vi "Build.vi"(6 "Type of Hexaboard":T1, 9 "XYZTheta":dbl[](array[numeric]), 10 "Pattern Coordinates":dbl[][](array[numeric]), 11 "C4 Dispense in":refnum<class "Iterative Dispense.lvclass">) -> (3 "C4 Dispense out":refnum<class "Iterative Dispense.lvclass">)   [LabVIEW 2021, in "Iterative Dispense.lvclass"]
uses:
  Iterative Dispense.lvclass
  C:/Users/hep/Documents/UCSB-CMU-GantryCode/UCSB-Gantry-HEP-main (3)/UCSB-Gantry-HEP-main/Classes/Routine/Dispense/Dispense.lvclass
  TypeOfHexaboard.ctl
  Iterative Dispense.lvclass/Iterative Dispense.ctl
  <vilib>/Analysis/coordinate.llb/2D Cartesian Coordinate Rotation (Array).vi
  <vilib>/Analysis/NI_AALPro.lvlib
  Routine.lvclass
panel:
  out "Array":dbl[][][](array[numeric])
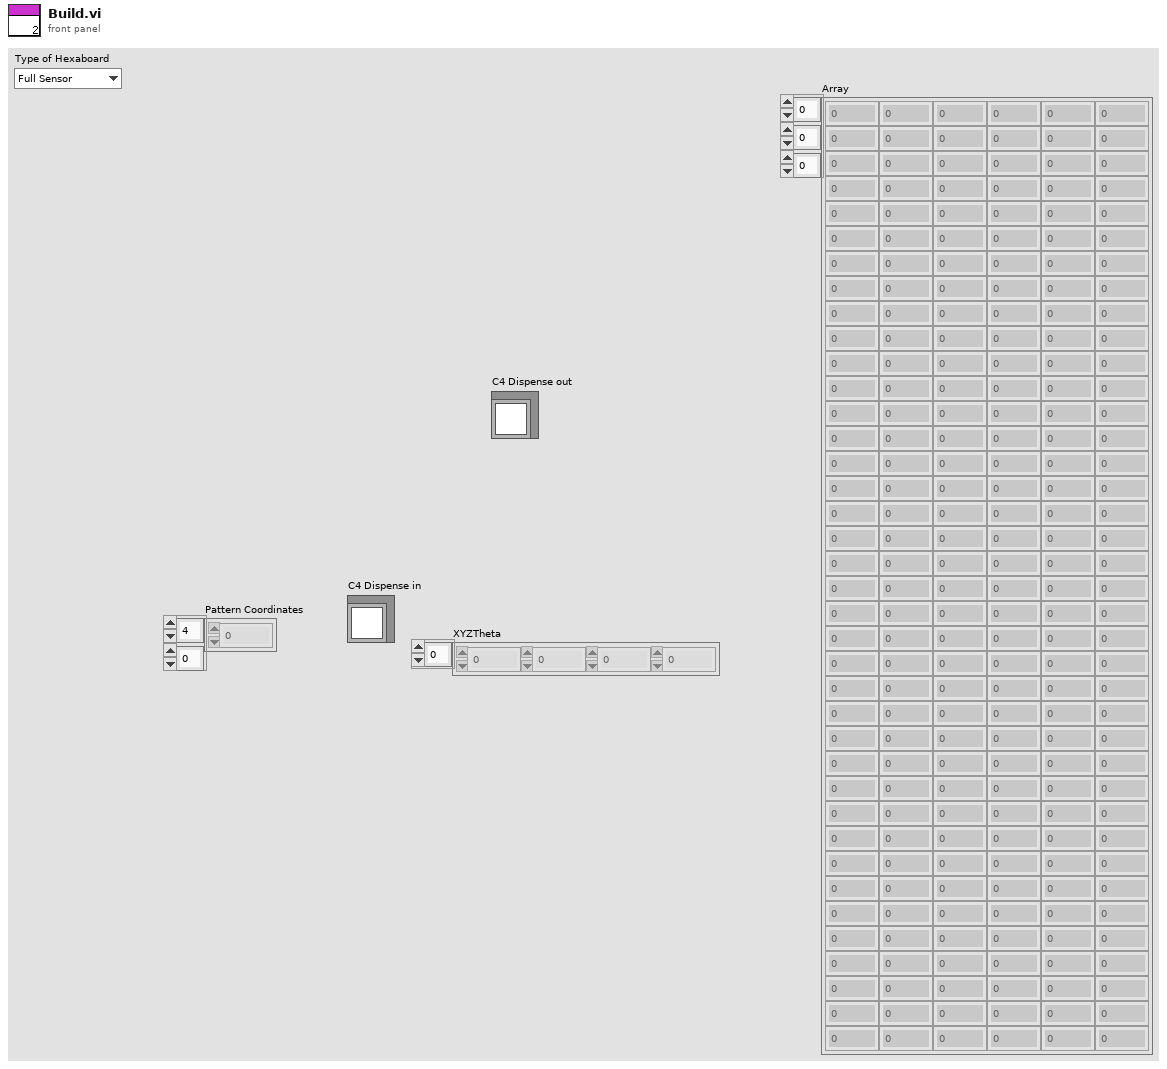
[diagram p1: front panel]
types:
  T1 = typedef "Routine.lvclass/TypeOfHexaboard.ctl" = enum16{"Full Sensor", "Full PCB", "Right Partial PCB", "Right Partial Sensor", "Al Dummy Right Partial Sensor"}
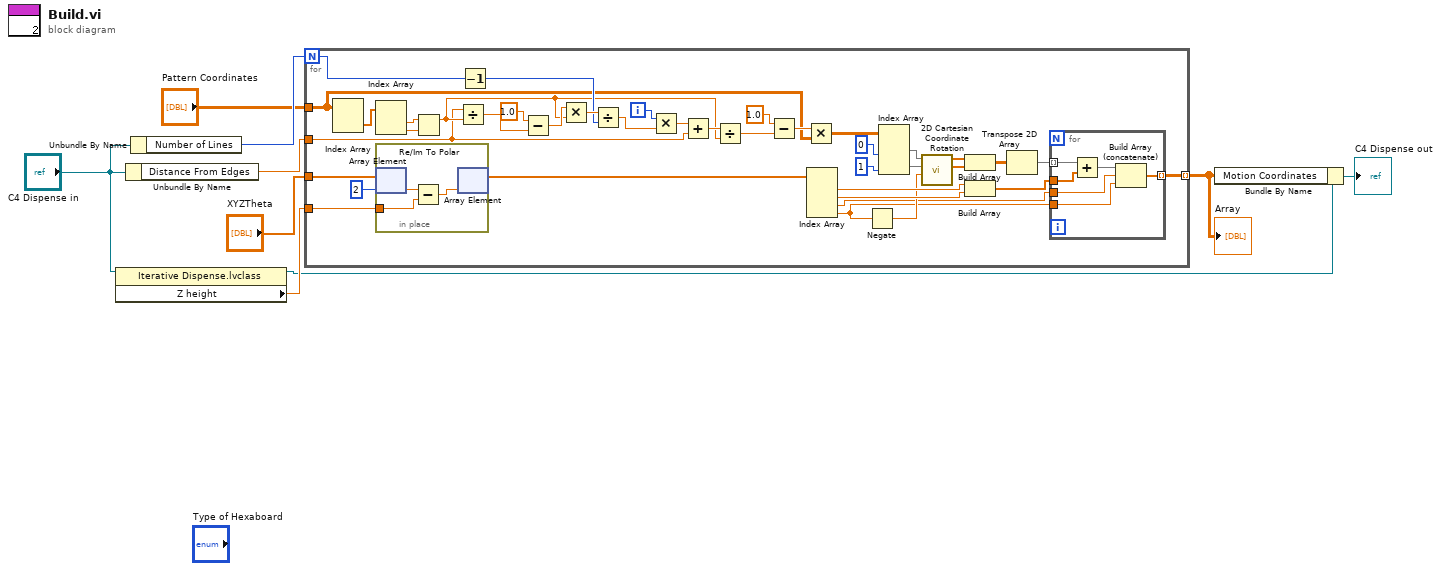
[diagram p0: block diagram]
diagram:
  n1 = property class="Iterative Dispense.lvclass"(reference="C4 Dispense in") -> (reference out=w3:refnum<class "Iterative Dispense.lvclass">, "Z height"=w7:dbl)  [unwired: 1 in, 1 out]
  n2 = Unbundle By Name("C4 Dispense in") -> ("Distance From Edges"=w6:dbl)
  n3 = Unbundle By Name("C4 Dispense in") -> ("Number of Lines"=w8:i32)
  n4 = for {
    N: w8 -> [w27]
    tunnel: "XYZTheta" -> [w16]
    tunnel: "Pattern Coordinates" -> [w24]
    tunnel: w7 -> [w15]
    tunnel: [w11] -> w2 mode=indexing
    tunnel: w6 -> [w10]
    i -> [w43]
    n5 = Index Array(array=w24) -> (element=w23:dbl[])  [unwired: 2 in]
    n6 = Index Array(array=w23) -> (element #1=w22:dbl, element #2=w21:dbl)  [unwired: 2 in]
    n7 = in-place {
      in-place-border: w15 -> [w50]
      n8 = in-place-array #1(w16, 2) -> (w51:dbl)
      n9 = Subtract(x=w51, y=w50) -> (x-y=w49:dbl)
      n10 = in-place-array #1(w49) -> (w14:dbl[])  [unwired: 1 out]
    }
    n11 = Re/Im To Polar(2:w21, 3:w22) -> (1:w31:dbl)  [unwired: 1 out]
    n12 = Divide(x=w10, y=w31) -> (x/y=w37:dbl)
    n13 = Decrement(x=w27) -> (x-1=w33:i32)
    n14 = Subtract(x=1.0, y=w37) -> (x-y=w35:dbl)
    n15 = Multiply(x=w35, y=w31) -> (x*y=w34:dbl)
    n16 = Divide(x=w34, y=w33) -> (x/y=w32:dbl)
    n17 = Multiply(x=w43, y=w32) -> (x*y=w48:dbl)
    n18 = Add(x=w48, y=w10) -> (x+y=w47:dbl)
    n19 = Divide(x=w47, y=w31) -> (x/y=w46:dbl)
    n20 = Subtract(x=1.0, y=w46) -> (x-y=w38:dbl)
    n21 = Multiply(x=w38, y=w24) -> (x*y=w44:dbl[][])
    n22 = Index Array(array=w14) -> (element #1=w30:dbl, element #2=w29:dbl, element #3=w13:dbl, element #4=w12:dbl)  [unwired: 4 in]
    n23 = Negate(x=w12) -> (-x=w18:dbl)
    n24 = Index Array(array=w44, index (col) #1=0 ("disabled index (col)"), index (col) #2=1 ("index (col)")) -> (element #1=w26:dbl[], element #2=w25:dbl[])  [unwired: 2 in]
    n25 = call-poly <vilib>:"2D Cartesian Coordinate Rotation.vi"("theta"=w18, "Y"=w25, "X"=w26) -> ("Y Out"=w42:dbl[], "X Out"=w41:dbl[])  [unwired: 6 in, 1 out]
    n26 = Build Array(w41, w42) -> (w20:dbl[][])
    n27 = Build Array(w30, w29) -> (w28:dbl[])
    n28 = Transpose 2D Array(2D array=w20) -> (transposed array=w19:dbl[][])
    n29 = for {
      tunnel: w28 -> [w57]
      tunnel: w19 -> [w56] mode=indexing
      tunnel: w13 -> [w54]
      tunnel: w12 -> [w53]
      tunnel: [w52] -> w11 mode=indexing
      n30 = Add(x=w56, y=w57) -> (x+y=w55:dbl[])
      n31 = Build Array (concatenate)(w55, w54, w53) -> (w52:dbl[])
    }
  }
  "Array" <- w2
  n32 = Bundle By Name(cluster=w3, "Motion Coordinates"=w2) -> (→"C4 Dispense out":refnum<class "Iterative Dispense.lvclass">)
